vi "ReadSetPoint.vi"(8 "error in (no error)":errorcluster, 10 "Port Number":u16=2000, 11 "IP Address":string="192.168.12.200") -> (0 "error out":errorcluster, 3 "Set Point":dbl format="%.2f")   [LabVIEW 2013, in "ovenCtrl.lvlib"]
uses:
  ovenCtrl.lvlib
panel:
  # "Inputs"
  # "Outputs"
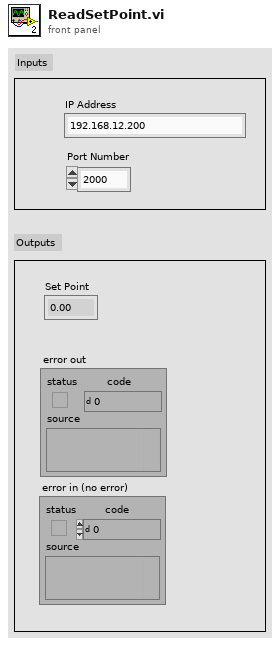
[diagram p1: front panel]
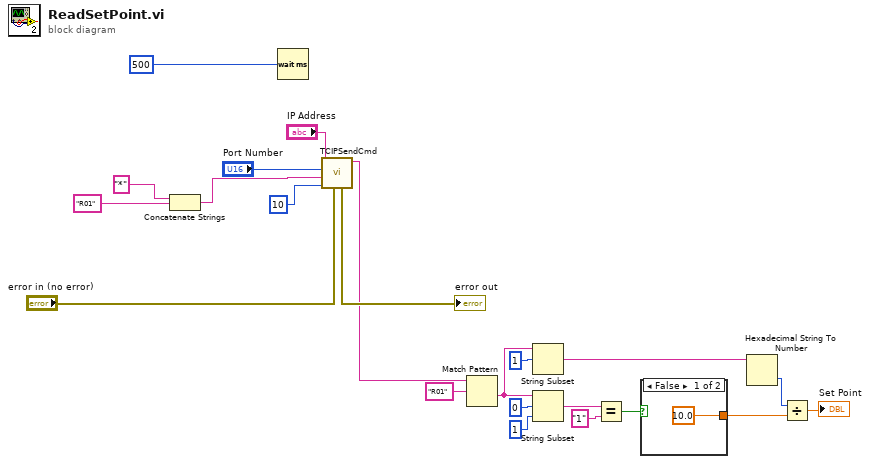
[diagram p0: block diagram]
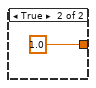
[diagram p2: hidden frame]
diagram:
  n1 = Concatenate Strings("*" ("string"), "R01" ("string")) -> (w17:string)
  n2 = Wait (ms)(milliseconds to wait=u32 500) -> ()  [unwired: 1 out]
  n3 = call "TCIPSendCmd.vi"("error in (no error)"="error in (no error)", "bytes to read"=10, "Command"=w17, "Port Number"="Port Number", "IP Address"="IP Address") -> ("Output Reading"=w1:string, "error out"=→"error out":errorcluster)  [unwired: 5 in]
  n4 = Match Pattern(string=w1, regular expression="R01") -> (after substring=w8:string)  [unwired: 1 in, 3 out]
  n5 = String Subset(string=w8, offset (0)=1) -> (substring=w6:string)  [unwired: 1 in]
  n6 = String Subset(string=w8, offset (0)=0, length (rest)=1) -> (substring=w5:string)
  n7 = Equal?(x=w5, y="1") -> (x = y?=w3:bool)
  n8 = case shown="False" w3 {
    tunnel: [10.0 1.0 ("y")] -> w2
    frame False {
    }
    frame True {
    }
  }
  n9 = Hexadecimal String To Number(string=w6) -> (number=w12:u32)  [unwired: 2 in, 1 out]
  n10 = Divide(x=w12, y=w2) -> (x/y=→"Set Point":dbl)
